vi "Launch On-Grid Actor for Testing.vi"   [LabVIEW 2016, in "On-Grid Actor.lvlib"]
uses:
  On-Grid Actor.lvlib
  On-Grid/On-Grid.lvclass
  C:/Users/Administrator/Desktop/LabVIEW EMS/EMS Generic Actor/EMS Generic/EMS Generic.lvclass
  C:/Program Files (x86)/National Instruments/LabVIEW 2016/vi.lib/ActorFramework/Actor/Actor.lvclass
  EMS Generic Actor/EMS Generic/Controls/Data Type DVRs.ctl
  EMS Generic Actor/EMS Generic/EMS Generic.lvclass/EMS Generic.ctl
  <vilib>/ActorFramework/Actor/Actor.lvclass
  EMS Generic Actor/EMS Generic/EMS Generic.lvclass
types:
  T1 = typedef "EMS Generic Actor.lvlib/EMS Generic.lvclass/Data Type DVRs.ctl" = cluster{"IED_Status":refnum<data-value>, "IED_Status_0":refnum<data-value>, "DER_Measurement":refnum<data-value>, "DER_Info":refnum<data-value>, "DER_Status":refnum<data-value>, "ES_Measurement":refnum<data-value>, "ES_Info":refnum<data-value>, "PV_Info":refnum<data-value>, "SmartRelay_Info":refnum<data-value>, "SmartRelay_Measurement":refnum<data-value>, "Meter_Info":refnum<data-value>, "Meter_Measurement":refnum<data-value>, "HVAC_Status":refnum<data-value>, "HVAC_Measurement":refnum<data-value>, "PriceData_RealTime":refnum<data-value>, "PriceData_Demand":refnum<data-value>, "PriceData_Energy":refnum<data-value>, "ForecastData_Long":refnum<data-value>, "ForecastData_Short":refnum<data-value>, "DER_Control":refnum<data-value>, "DER_SetPointF":refnum<data-value>, "DER_SetPointP":refnum<data-value>, "DER_SetPointQ":refnum<data-value>, "DER_SetPointPF":refnum<data-value>, "DER_SetPointV":refnum<data-value>, "PV_setCurtailment":refnum<data-value>, "PV_setRampRate":refnum<data-value>, "Relay_Control":refnum<data-value>, "Load_Control":refnum<data-value>, "HVAC_Control":refnum<data-value>, "Generator_Info":refnum<data-value>, "ForecastData_Long_Backup":refnum<data-value>, "PriceData_RealTime_Backup":refnum<data-value>}
  T2 = cluster{"[0]":refnum<data-value>, "[1]":refnum<data-value>, "[2]":refnum<data-value>, "[3]":refnum<data-value>, "[4]":refnum<data-value>, "[5]":refnum<data-value>, "[6]":refnum<data-value>, "[7]":refnum<data-value>, "[8]":refnum<data-value>, "[9]":refnum<data-value>, "[10]":refnum<data-value>, "[11]":refnum<data-value>, "[12]":refnum<data-value>, "[13]":refnum<data-value>, "[14]":refnum<data-value>, "[15]":refnum<data-value>, "[16]":refnum<data-value>, "[17]":refnum<data-value>, "[18]":refnum<data-value>, "[19]":refnum<data-value>, "[20]":refnum<data-value>, "[21]":refnum<data-value>, "[22]":refnum<data-value>, "[23]":refnum<data-value>, "[24]":refnum<data-value>, "[25]":refnum<data-value>, "[26]":refnum<data-value>, "[27]":refnum<data-value>, "[28]":refnum<data-value>, "[29]":refnum<data-value>}
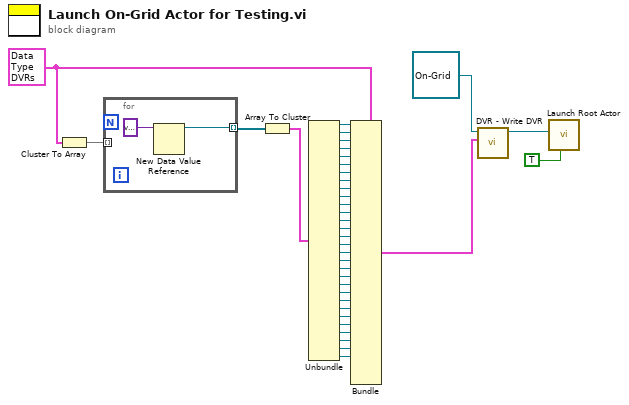
[diagram p0: block diagram]
diagram:
  w34 = T1 {"IED_Status"=refnum, "IED_Status_0"=refnum, "DER_Measurement"=refnum, "DER_Info"=refnum, "DER_Status"=refnum, "ES_Measurement"=refnum, "ES_Info"=refnum, "PV_Info"=refnum, "SmartRelay_Info"=refnum, "SmartRelay_Measurement"=refnum, "Meter_Info"=refnum, "Meter_Measurement"=refnum, "HVAC_Status"=refnum, "HVAC_Measurement"=refnum, "PriceData_RealTime"=refnum, "PriceData_Demand"=refnum, "PriceData_Energy"=refnum, "ForecastData_Long"=refnum, "ForecastData_Short"=refnum, "DER_Control"=refnum, "DER_SetPointF"=refnum, "DER_SetPointP"=refnum, "DER_SetPointQ"=refnum, "DER_SetPointPF"=refnum, "DER_SetPointV"=refnum, "PV_setCurtailment"=refnum, "PV_setRampRate"=refnum, "Relay_Control"=refnum, "Load_Control"=refnum, "HVAC_Control"=refnum, "Generator_Info"=refnum, "ForecastData_Long_Backup"=refnum, "PriceData_RealTime_Backup"=refnum} ("DVR")
  n1 = Cluster To Array(cluster=w34) -> (array=w37:refnum<data-value>[])
  n2 = for {
    tunnel: w37 -> [_] mode=indexing
    tunnel: [w39] -> w36 mode=indexing
    n3 = New Data Value Reference(data value=variant ("data")) -> (data value reference=w39:refnum<data-value>)  [unwired: 1 in, 1 out]
  }
  n4 = Array To Cluster(array=w36) -> (cluster=w35:T2)
  n5 = Unbundle(w35) -> ("[0]"=w33:refnum<data-value>, "[1]"=w32:refnum<data-value>, "[2]"=w31:refnum<data-value>, "[3]"=w30:refnum<data-value>, "[4]"=w29:refnum<data-value>, "[5]"=w28:refnum<data-value>, "[6]"=w27:refnum<data-value>, "[7]"=w26:refnum<data-value>, "[8]"=w25:refnum<data-value>, "[9]"=w24:refnum<data-value>, "[10]"=w23:refnum<data-value>, "[11]"=w22:refnum<data-value>, "[12]"=w21:refnum<data-value>, "[13]"=w20:refnum<data-value>, "[14]"=w19:refnum<data-value>, "[15]"=w18:refnum<data-value>, "[16]"=w17:refnum<data-value>, "[17]"=w16:refnum<data-value>, "[18]"=w15:refnum<data-value>, "[19]"=w14:refnum<data-value>, "[20]"=w13:refnum<data-value>, "[21]"=w12:refnum<data-value>, "[22]"=w11:refnum<data-value>, "[23]"=w10:refnum<data-value>, "[24]"=w9:refnum<data-value>, "[25]"=w8:refnum<data-value>, "[26]"=w7:refnum<data-value>, "[27]"=w6:refnum<data-value>, "[28]"=w2:refnum<data-value>, "[29]"=w1:refnum<data-value>)
  n6 = Bundle(cluster=w34, "IED_Status"=w33, "IED_Status_0"=w32, "DER_Measurement"=w31, "DER_Info"=w30, "DER_Status"=w29, "ES_Measurement"=w28, "ES_Info"=w27, "PV_Info"=w26, "SmartRelay_Info"=w25, "SmartRelay_Measurement"=w24, "Meter_Info"=w23, "Meter_Measurement"=w22, "HVAC_Status"=w21, "HVAC_Measurement"=w20, "PriceData_RealTime"=w19, "PriceData_Demand"=w18, "PriceData_Energy"=w17, "ForecastData_Long"=w16, "ForecastData_Short"=w15, "DER_Control"=w14, "DER_SetPointF"=w13, "DER_SetPointP"=w12, "DER_SetPointQ"=w11, "DER_SetPointPF"=w10, "DER_SetPointV"=w9, "PV_setCurtailment"=w8, "PV_setRampRate"=w7, "Relay_Control"=w6, "Load_Control"=w2, "HVAC_Control"=w1) -> (w3:T1)  [unwired: 3 in]
  n7 = call "DVR - Write DVR.vi"("DVR"=w3, "EMS Generic in"=refnum<class "On-Grid.lvclass"> refnum ("On-Grid Actor.lvlib:On-Grid.lvclass")) -> ("EMS Generic out"=w4:refnum<class "On-Grid.lvclass">)  [unwired: 9 in]
  n8 = call <vilib>:"Launch Root Actor.vi"("Open Actor Core front panel? (F)"=TRUE, "Actor"=w4) -> ()  [unwired: 8 in, 2 out]
